vi "APITemplateRequest.vi"(6 "Instance":i32) -> ()   [LabVIEW 2017, in "Communication.lvlib"]
uses:
  Communication.lvlib
panel:
  out "error out":errorcluster
  in  "error in (no error)":errorcluster
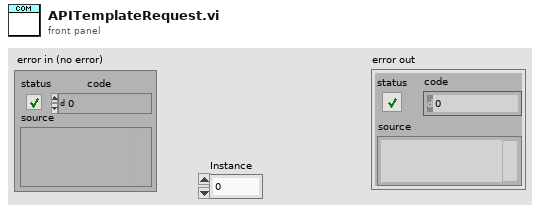
[diagram p1: front panel]
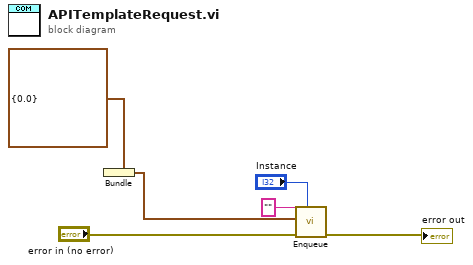
[diagram p0: block diagram]
diagram:
  n1 = Bundle(cluster=cluster{dbl} {0.0}) -> (w2:cluster{dbl})  [unwired: 1 in]
  n2 = call "Enqueue.vi"("Instance"="Instance", "error in (no error)"="error in (no error)", "Data"=w2, "Msg"="") -> ("error out"=→"error out":errorcluster)  [unwired: 7 in]
